vi "Mass Compile - UI - .vi"(7 "Only Check Launcher? (F: Check Entire Product)":bool, 8 "error in (no error)":errorcluster, 10 "Product Folders":path[](array[path]), 11 "Product Name":string) -> (0 "error out":errorcluster, 2 "User Aborted?":bool)   [LabVIEW 2013]
uses:
  <userlib>/_OpenG.lib/appcontrol/appcontrol.llb/Close Generic Object Refnum (Array VI)__ogtk.vi
  <userlib>/_OpenG.lib/array/array.llb/Conditional Auto-Indexing Tunnel (VI-REF)__ogtk.vi
  <userlib>/_OpenG.lib/array/array.llb/Conditional Auto-Indexing Tunnel (Variant)__ogtk.vi
  <userlib>/_OpenG.lib/array/array.llb/Remove Duplicates from 1D Array (String)__ogtk.vi
  <userlib>/_OpenG.lib/array/array.llb/Delete Elements from 1D Array (Variant)__ogtk.vi
  <userlib>/_OpenG.lib/appcontrol/appcontrol.llb/Close Generic Object Refnum (Scalar VI)__ogtk.vi
panel:
  out "Sub-state":string
  out "Slide":u8(slide) scale=0.0..100.0
  out "Elapsed Time":dbl format="%<%H:%M:%S%0u>t"
  in  "abort":bool
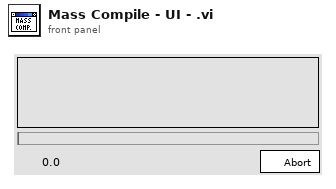
[diagram p1: front panel]
types:
  T1 = cluster{"Current VI's reference":refnum<vi>, "VIs to Recompiled":refnum<vi>[], "Libraries to Recompiled":refnum<vi>[], "Total size":i32, "Current":i32, "Start time":timestamp, "VI Path":path, "Product Folders":path[], "User Aborted":bool}
  T2 = cluster{"Minimum":dbl, "Maximum":dbl, "Increment":dbl, "Minor Incr":dbl, "Start":dbl}
  T3 = enum32{"Invalid", "Standard", "Closed", "Hidden", "Minimized", "Maximized"}
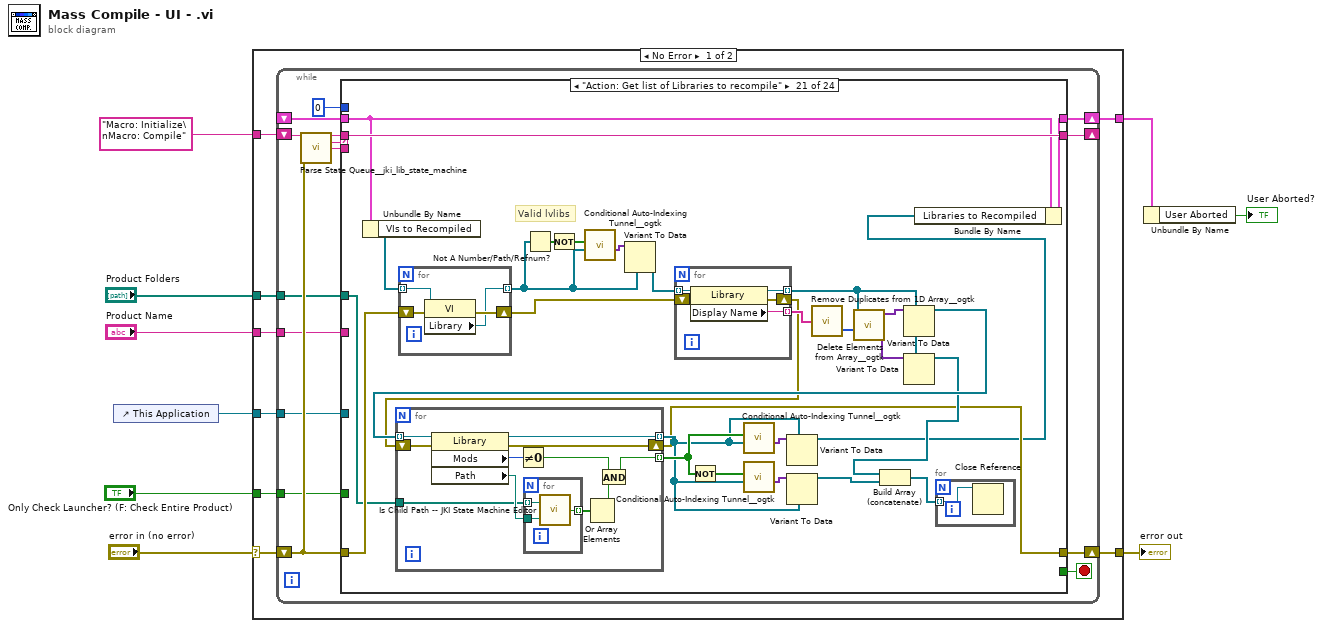
[diagram p0: block diagram]
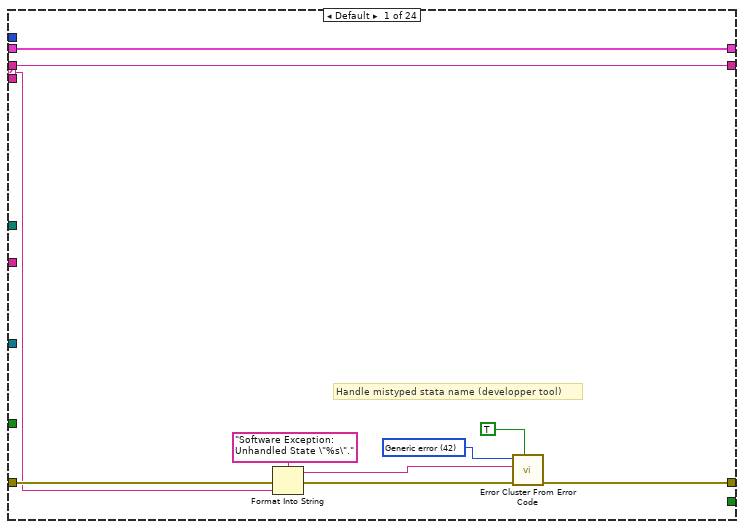
[diagram p2: hidden frame]
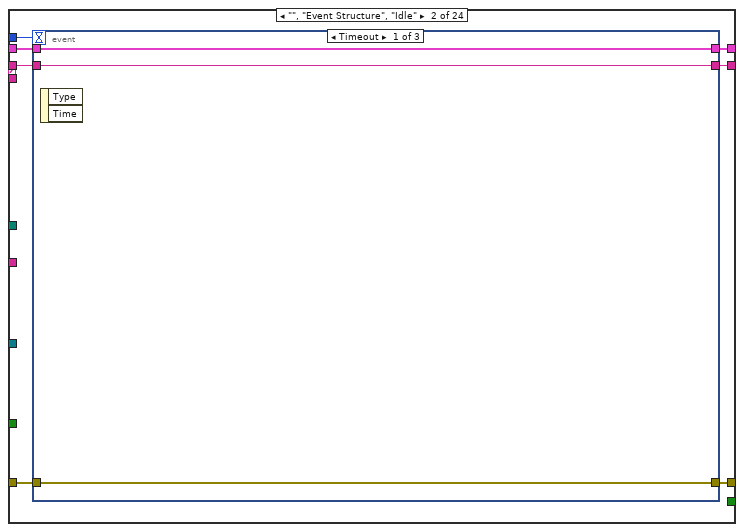
[diagram p3: hidden frame]
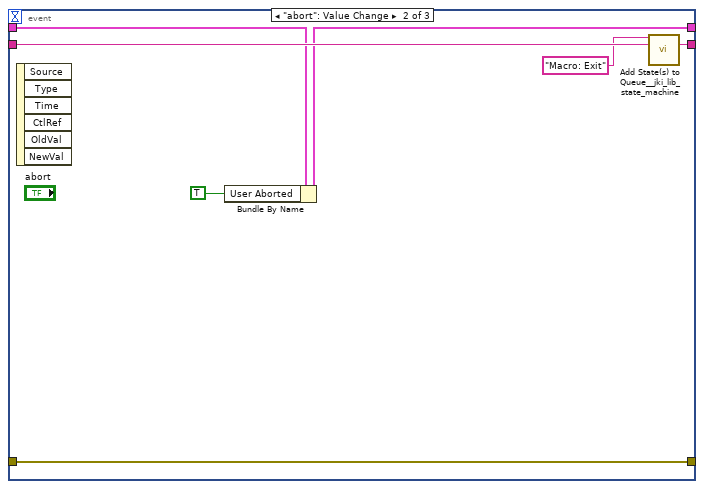
[diagram p4: hidden frame]
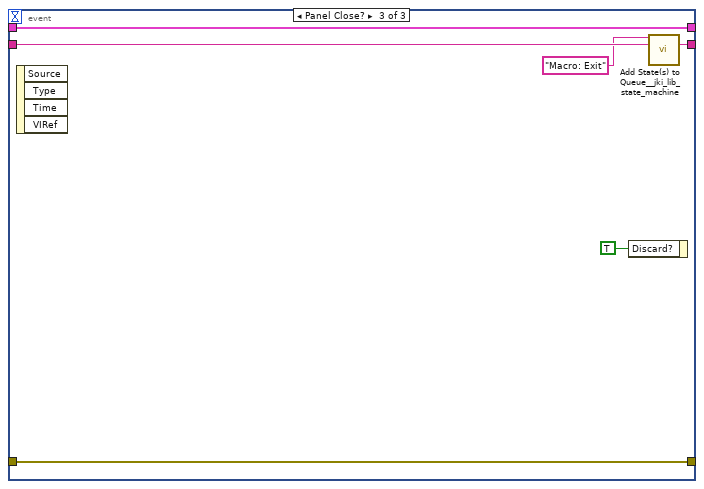
[diagram p5: hidden frame]
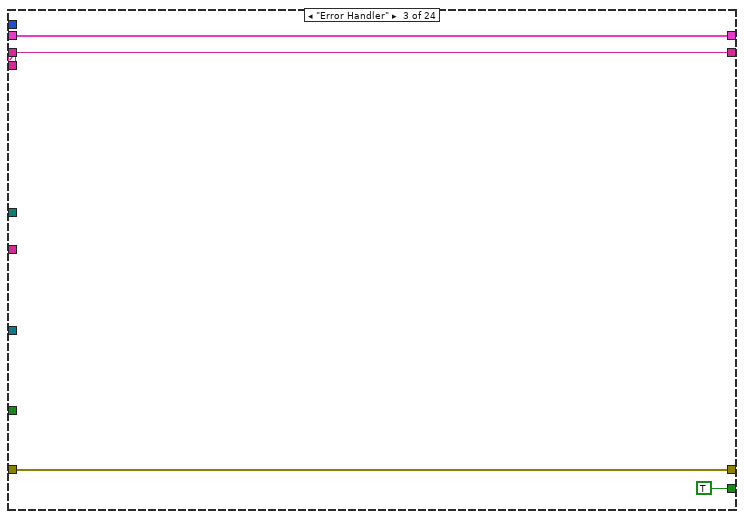
[diagram p6: hidden frame]
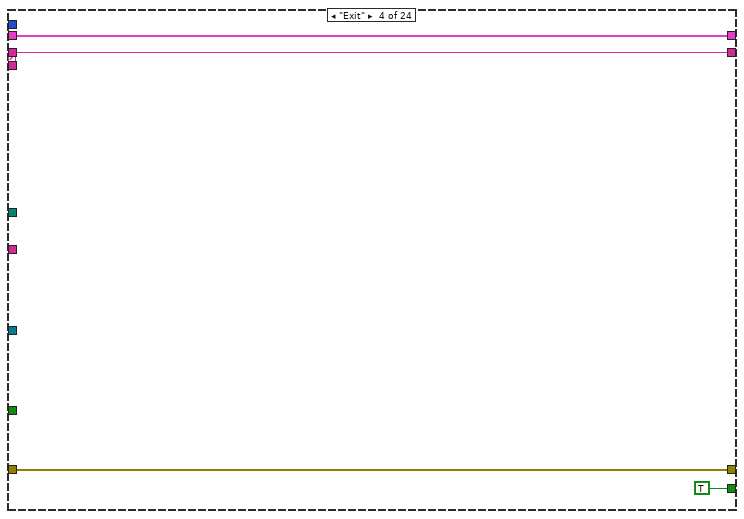
[diagram p7: hidden frame]
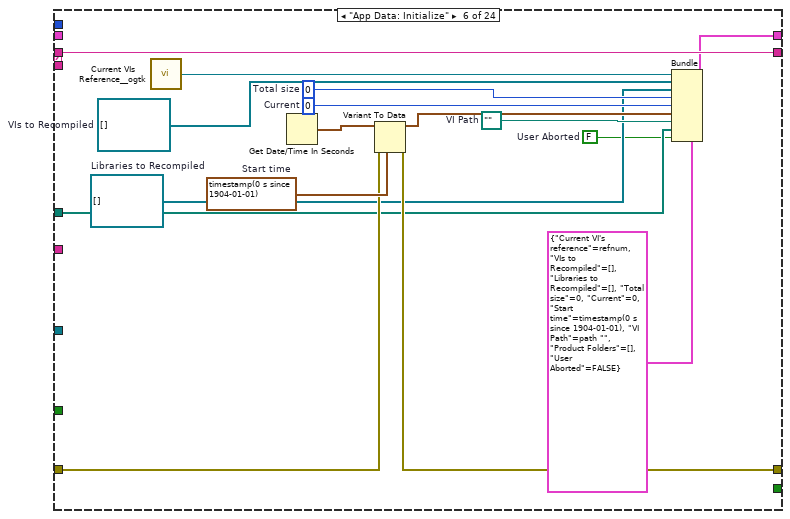
[diagram p9: hidden frame]
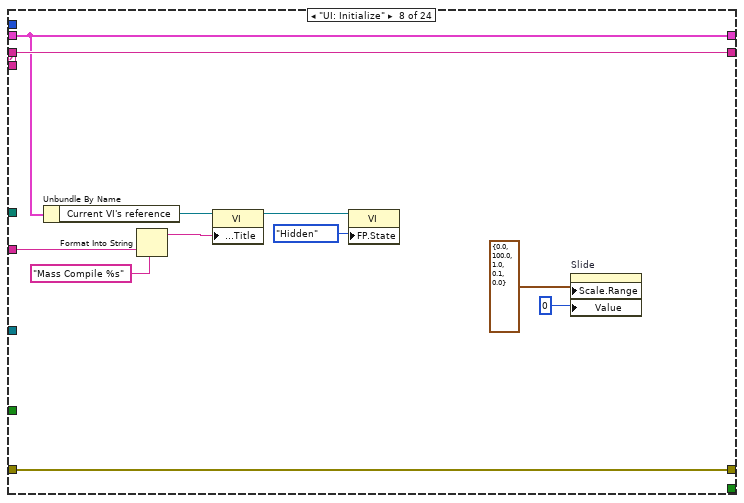
[diagram p11: hidden frame]
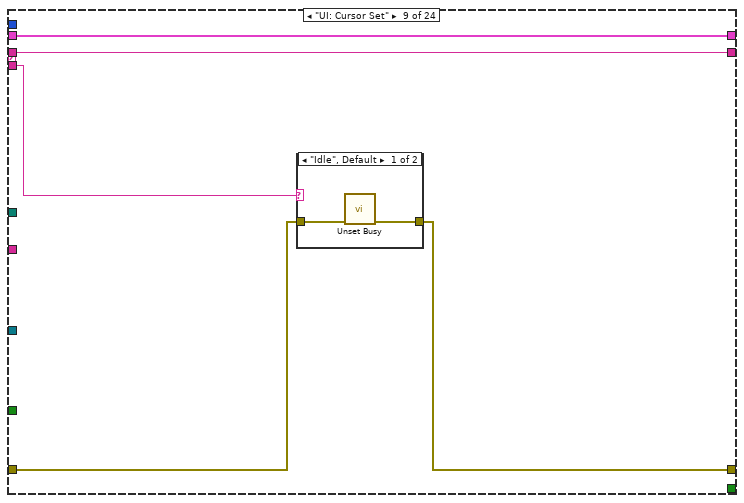
[diagram p12: hidden frame]
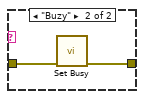
[diagram p13: hidden frame]
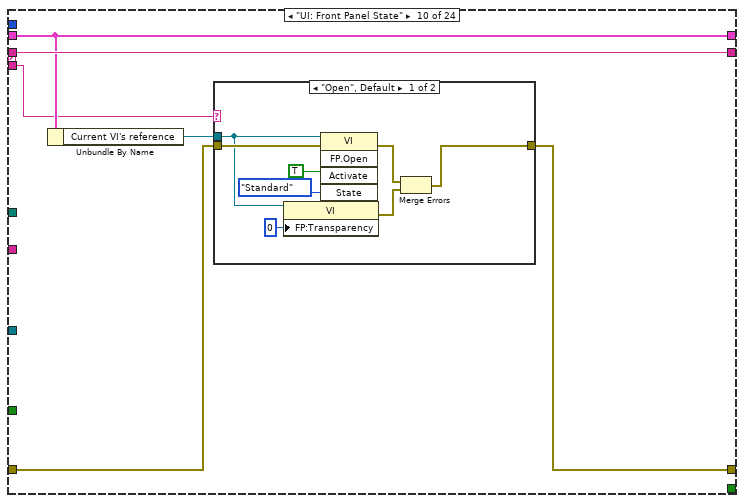
[diagram p14: hidden frame]
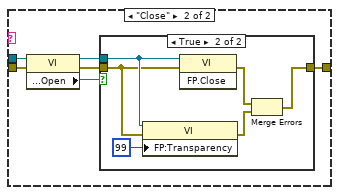
[diagram p15: hidden frame]
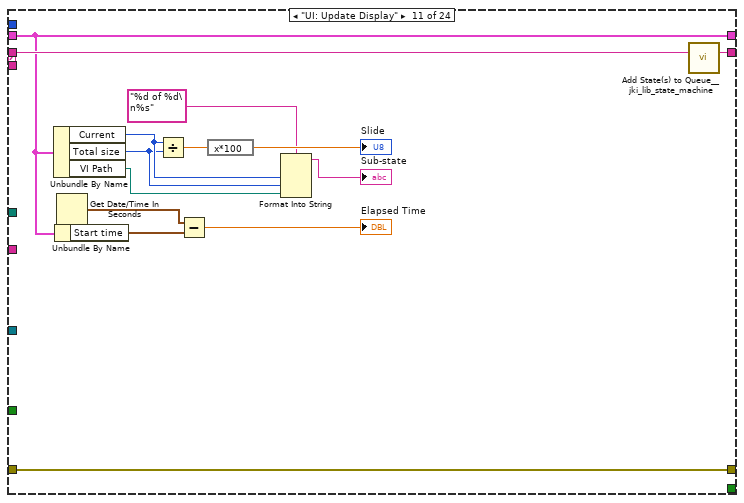
[diagram p17: hidden frame]
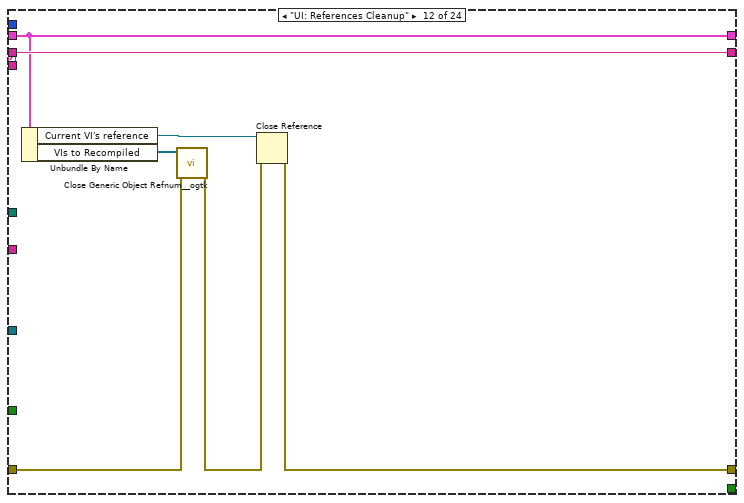
[diagram p18: hidden frame]
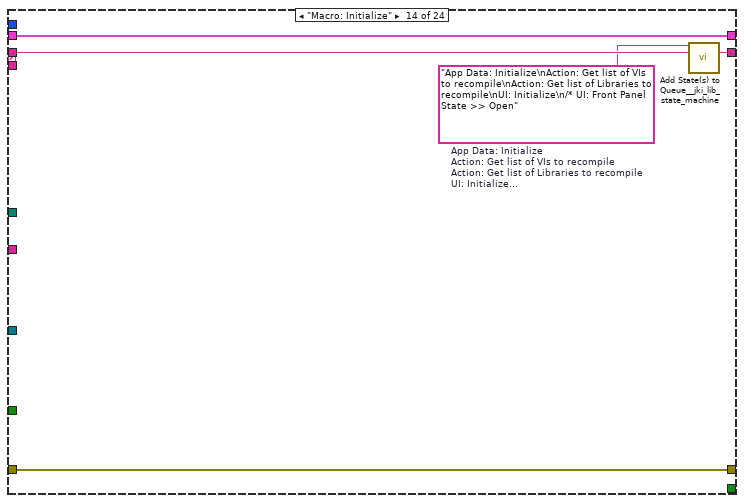
[diagram p20: hidden frame]
diagram:
  n1 = control-ref of="This Application"() -> (w3:refnum<vi>)
  n2 = case shown="No Error" "error in (no error)" {
    selector: "error in (no error)" -> [w14 w365]
    tunnel: "Macro: Initialize\nMacro: Compile" -> [w17 _]
    tunnel: "Product Name" -> [w16 _]
    tunnel: [w15 w365] -> w7
    tunnel: "Product Folders" -> [w13 _]
    tunnel: "Only Check Launcher? (F: Check Entire Product)" -> [w12 _]
    tunnel: w3 -> [w11 _]
    tunnel: [w10 _] -> w2
    frame No Error {
      n3 = while {
        shift-right: [w23] -> w10
        shift-left: _ -> [w28]
        shift-right: [w27] -> w15
        shift-left: w14 -> [w26]
        shift-right: [w25] -> _
        shift-left: w17 -> [w29]
        tunnel: w16 -> [w22]
        tunnel: w13 -> [w20]
        tunnel: w12 -> [w19]
        tunnel: w11 -> [w18]
        stop <- w24 stop-if-true
        n4 = call <vilib>:"Parse State Queue__jki_lib_state_machine.vi"("State Queue"=w29, "Error In (no error)"=w26) -> ("Remaining States"=w31:string, "Current State"=w32:string, "Arguments"=w30:string)  [unwired: 11 in]
        n5 = case shown="\"Action: Get list of Libraries to recompile\"" w32 {
          selector: w32 -> [w36 _ _ _ _ _ _ _ _ _ _ _ _ _ _ _ _ _ _ _ _ _ w332 _]
          tunnel: w31 -> [w35 w49 w69 w73 w76 w92 w95 w106 w111 w121 w156 w163 w166 w171 w190 w201 w204 w209 w219 w239 w299 w329 w354 w359]
          tunnel: w30 -> [_ _ _ _ _ _ _ _ w107 w118 _ _ _ _ _ _ _ _ _ _ _ w327 _ _]
          tunnel: w28 -> [w34 w47 w68 w72 w74 _ w93 w105 w110 w119 w152 w162 w164 w168 w187 w198 w202 w206 w217 w234 w289 w328 w342 w358]
          tunnel: [w38 w46 w67 w71 w75 w82 w94 w96 w108 w116 w148 w160 w165 w169 w188 w199 w203 w207 w218 w231 w272 w325 w351 w356] -> w27
          tunnel: w26 -> [w37 w45 w67 w71 w75 w83 w94 w96 w109 w117 w148 w158 w165 w169 w188 w199 w203 w207 w218 w232 w287 w326 w343 w355]
          tunnel: [w35 w48 w69 w73 w76 w92 w95 w106 w111 w121 w155 w163 w166 w170 w189 w200 w204 w208 w219 w239 w299 w329 w353 w359] -> w25
          tunnel: [_ _ TRUE TRUE _ _ _ _ _ _ _ _ _ _ _ _ _ _ _ _ _ _ _ _] -> w24
          tunnel: [w34 w44 w68 w72 w74 w91 w93 w105 w110 w119 w152 w162 w164 w168 w187 w198 w202 w206 w217 w233 w298 w328 w352 w358] -> w23
          tunnel: w22 -> [_ _ _ _ _ _ _ w98 _ _ _ _ _ _ w182 _ _ _ _ _ _ _ _ _]
          tunnel: 0 -> [_ w43 _ _ _ _ _ _ _ _ _ _ _ _ _ _ _ _ _ _ _ _ _ _]
          tunnel: w20 -> [_ _ _ _ _ w80 _ _ _ _ _ _ _ _ _ _ _ _ _ w229 w277 _ _ _]
          tunnel: w19 -> [_ _ _ _ _ _ _ _ _ _ _ _ _ _ _ _ _ _ _ w220 _ _ _ _]
          tunnel: w18 -> [_ _ _ _ _ _ _ _ _ _ _ _ _ _ _ _ _ _ _ w221 _ _ _ _]
          frame Default {
            w41 = 42 items=["No error", "Argument error", "Memory is full", "Out of zone", "End of file", "File already open", "Generic file I/O error", "File not found", "File permission error", "Disk is full", "Duplicate path", "Too many files open", "System feature not enabled", "Resource file not found", "Cannot add resource", "Resource not found", "Image not found", "Image memory error", "Pen does not exist", "Config type invalid", "Config token not found", "Config parse error", "Config memory error", "Bad external code format", "Bad external code offset", "External code not present", "Null window", "Destroy window error", "Null menu", "Print aborted", "Bad print record", "Print driver error", "Windows error during printing", "Memory error during printing", "Print dialog error", "Generic print error", "Invalid device refnum", "Device not found", "Device parameter error", "Device unit error", "Cannot open device", "Device call aborted", "Generic error", "Cancelled by user", "Object ID too low", "Object ID too high", "Object not in heap", "Unknown heap", "Unknown object (invalid DefProc)", "Unknown object (DefProc not in table)", "Message out of range", "Invalid (null) method", "Unknown message", "Manager call not supported", "Bad address", "Network operation in progress", "Network operation timed out", "Connection is busy", "Network attribute not supported", "Network error", "Address in use", "System out of memory", "Connection aborted", "Connection refused", "Not connected", "Already connected", "Connection closed", "Initialization error (interapplication manager)", "Bad occurrence", "Wait on unbound occurrence handler", "Occurrence queue overflow", "Datalog type conflict", "Unused", "Unrecognized type (interapplication manager)", "Memory corrupt", "Failed to make temporary DLL", "Old CIN version", "Drag socket not found", "Failed to load drop-object", "Failed to register OLE object", "Failed to release OLE object", "Format specifier type mismatch", "Unknown format specifier", "Too few format specifiers", "Too many format specifiers", "Scan failed", "Newer CIN version", "Error converting to variant", "Runtime menu error", "Password tampered", "Variant attribute not found", "Incompatible variant data type", "Event data is not available", "Event Store is not present", "Occurrence is not found", "Event Queue is not created", "Event info is not available", "Refnum passed is NULL", "Error retrieving Class GUID", "Error retrieving CoClass GUID", "Error retrieving TypeLib GUID.", "Bad built application magic bytes.", "Specific driver is different from the specific driver associated with the Logical Name.", "There is no session opened to the class driver.", "Max Error", "MAX - Error with config objects", "MAX - Error loading configuration", "MAX - Group not supported"]
            # "Handle mistyped stata name (developper tool)"
            n6 = Format Into String(format string="Software Exception: Unhandled State \"%s\"." ("message"), error in=w37, w36) -> (resulting string=w40:string, error out=w39:errorcluster)  [unwired: 1 in]
            n7 = call <vilib>:"Error Cluster From Error Code.vi"("show call chain? (False)"=TRUE, "error in (no error)"=w39, "error message (\"\")"=w40, "error code (0)"=w41) -> ("error out"=w38:errorcluster)  [unwired: 5 in]
          }
          frame "", "Event Structure", "Idle" {
            n8 = event shown="[0] Timeout" {
              selector: _ -> [_ _ _]
              dyn-events: _ -> [_ _ _]
              timeout: w43 -> [_ _ _]
              tunnel: w49 -> [w52 w59 w65]
              tunnel: [w52 w58 w64] -> w48
              tunnel: w47 -> [w50 w56 w62]
              tunnel: [w51 w57 w63] -> w46
              tunnel: w45 -> [w51 w57 w63]
              tunnel: [w50 w54 w62] -> w44
              event Timeout {
                n9 = event-data() -> ()  [unwired: 1 in, 2 out]
              }
              event "abort": Value Change {
                n10 = event-data() -> ()  [unwired: 1 in, 6 out]
                n11 = Bundle By Name(cluster=w56, "User Aborted"=TRUE) -> (w54:T1)
                n12 = call <vilib>:"Add State(s) to Queue__jki_lib_state_machine.vi"("State(s) in Front (\"\")"="Macro: Exit", "State(s) in (\"\")"=w59) -> ("States Out"=w58:string)  [unwired: 13 in]
              }
              event Panel Close? {
                n13 = event-data() -> ()  [unwired: 1 in, 4 out]
                n14 = event-data("Discard?"=TRUE) -> ()  [unwired: 1 in, 1 out]
                n15 = call <vilib>:"Add State(s) to Queue__jki_lib_state_machine.vi"("State(s) in Front (\"\")"="Macro: Exit", "State(s) in (\"\")"=w65) -> ("States Out"=w64:string)  [unwired: 13 in]
              }
            }
          }
          frame "Error Handler" {
          }
          frame "Exit" {
          }
          frame "---------- App Data ----------" {
          }
          frame "App Data: Initialize" {
            w77 = FALSE  # User Aborted
            w79 = refnum<vi>[] []  # Libraries to Recompiled
            w81 = path ""  # VI Path
            w86 = timestamp(0 s since 1904-01-01)  # Start time
            w87 = 0  # Current
            w88 = 0  # Total size
            w89 = refnum<vi>[] []  # VIs to Recompiled
            n16 = call <userlib>:"Current VIs Reference__ogtk.vi"() -> ("Current VI's reference"=w90:refnum<vi>)  [unwired: 5 in]
            n17 = Get Date/Time In Seconds() -> (seconds since 1Jan1904=w85:timestamp)
            n18 = Variant To Data(error in=w83, type=w86, Variant=w85) -> (data=w84:timestamp, error out=w82:errorcluster)
            n19 = Bundle(cluster=T1 {"Current VI's reference"=refnum, "VIs to Recompiled"=[], "Libraries to Recompiled"=[], "Total size"=0, "Current"=0, "Start time"=timestamp(0 s since 1904-01-01), "VI Path"=path "", "Product Folders"=[], "User Aborted"=FALSE}, "Current VI's reference"=w90, "VIs to Recompiled"=w89, "Libraries to Recompiled"=w79, "Total size"=w88, "Current"=w87, "Start time"=w84, "VI Path"=w81, "Product Folders"=w80, "User Aborted"=w77) -> (w91:T1)
          }
          frame "---------- UI ----------" {
          }
          frame "UI: Initialize" {
            n20 = Unbundle By Name(w105) -> ("Current VI's reference"=w101:refnum<vi>)
            n21 = Format Into String(format string="Mass Compile %s", w98) -> (resulting string=w97:string)  [unwired: 2 in, 1 out]
            n22 = property class="VI"(reference=w101, "Front Panel.Title"=w97) -> (reference out=w100:refnum<vi>)  [unwired: 1 in, 1 out]
            n23 = property class="VI"(reference=w100, "FP.State"=T3."Hidden" ("Front Panel Window:State")) -> ()  [unwired: 1 in, 2 out]
            n24 = property on="Slide" class="Slide (strict)"("Scale.Range"=T2 {"Minimum"=0.0, "Maximum"=100.0, "Increment"=1.0, "Minor Incr"=0.1, "Start"=0.0}, "Value"=0) -> ()  [unwired: 2 in, 2 out]
          }
          frame "UI: Cursor Set" {
            n25 = case shown="\"Idle\", Default" w107 {
              tunnel: w109 -> [w113 w115]
              tunnel: [w112 w114] -> w108
              frame "Idle", Default {
                n26 = call <vilib>:"Unset Busy.vi"("error in (no error)"=w113) -> ("error out"=w112:errorcluster)  [unwired: 10 in]
              }
              frame "Buzy" {
                n27 = call <vilib>:"Set Busy.vi"("error in (no error)"=w115) -> ("error out"=w114:errorcluster)  [unwired: 9 in, 1 out]
              }
            }
          }
          frame "UI: Front Panel State" {
            n28 = Unbundle By Name(w119) -> ("Current VI's reference"=w120:refnum<vi>)
            n29 = case shown="\"Open\", Default" w118 {
              tunnel: w120 -> [w125 w134]
              tunnel: w117 -> [w127 w133]
              tunnel: [w122 w135] -> w116
              frame "Open", Default {
                n30 = property class="VI"(reference=w125, "FP:Transparency"=u8 0 ("Front Panel Window:Transparency")) -> (error out=w124:errorcluster)  [unwired: 1 in, 1 out]
                n31 = invoke class="VI" method="FP.Open"(reference=w125, error in=w127, "Activate"=TRUE, "State"=T3."Standard") -> (error out=w123:errorcluster)  [unwired: 1 in, 4 out]
                n32 = Merge Errors(w123, w124) -> (w122:errorcluster)
              }
              frame "Close" {
                n33 = property class="VI"(reference=w134, error in=w133) -> (reference out=w132:refnum<vi>, error out=w131:errorcluster, "Front Panel.Open"=w130:bool)
                n34 = case shown="True" w130 {
                  tunnel: w132 -> [_ w142]
                  tunnel: w131 -> [w136 w140]
                  tunnel: [w136 w137] -> w135
                  frame False {
                  }
                  frame True {
                    n35 = property class="VI"(reference=w142, error in=w140, "FP:Transparency"=u8 99 ("Front Panel Window:Transparency")) -> (error out=w138:errorcluster)  [unwired: 1 out]
                    n36 = invoke class="VI" method="FP.Close"(reference=w142, error in=w140) -> (error out=w139:errorcluster)  [unwired: 1 in, 2 out]
                    n37 = Merge Errors(w139, w138) -> (w137:errorcluster)
                  }
                }
              }
            }
          }
          frame "UI: Update Display" {
            n38 = Unbundle By Name(w152) -> ("Current"=w146:i32, "Total size"=w145:i32, "VI Path"=w144:path)
            n39 = Unbundle By Name(w152) -> ("Start time"=w151:timestamp)
            n40 = Get Date/Time In Seconds() -> (seconds since 1Jan1904=w150:timestamp)
            n41 = Divide(x=w146, y=w145) -> (x/y=w154:dbl)
            n42 = Subtract(x=w150, y=w151) -> (x-y=→"Elapsed Time":dbl)
            n43 = expression code="x*100"(w154) -> (→"Slide":dbl)
            n44 = Format Into String(format string="%d of %d\n%s", w146, w145, w144) -> (resulting string=→"Sub-state":string)  [unwired: 2 in, 1 out]
            n45 = call <vilib>:"Add State(s) to Queue__jki_lib_state_machine.vi"("State(s) in (\"\")"=w156) -> ("States Out"=w155:string)  [unwired: 14 in]
          }
          frame "UI: References Cleanup" {
            n46 = Unbundle By Name(w162) -> ("Current VI's reference"=w161:refnum<vi>, "VIs to Recompiled"=w159:refnum<vi>[])
            n47 = call-poly <userlib>:"Close Generic Object Refnum__ogtk.vi"("error in (no error)"=w158, "Gen Refnum Array"=w159) -> ("error out"=w157:errorcluster)  [unwired: 8 in, 1 out]
            n48 = Close Reference(reference=w161, error in (no error)=w157) -> (error out=w160:errorcluster)
          }
          frame "---------- Macro ----------" {
          }
          frame "Macro: Initialize" {
            w167 = "App Data: Initialize\nAction: Get list of VIs to recompile\nAction: Get list of Libraries to recompile\nUI: Initialize\n/* UI: Front Panel State >> Open"  # App Data: Initialize Action: Get list of VIs to recompile Action: Get list of Libraries to recompile UI: Initialize /* UI: Front Panel State >> Open
            n49 = call <vilib>:"Add State(s) to Queue__jki_lib_state_machine.vi"("State(s) in Front (\"\")"=w167, "State(s) in (\"\")"=w171) -> ("States Out"=w170:string)  [unwired: 13 in]
          }
          frame "Macro: Compile" {
            (unwired) "<color=red>You appears to be running the %s for the first time after installation. \nYou should mass compile the %s before you can use it effectively.</color>"
            w184 = "UI: Front Panel State >> Open\nAction: Set LLB Caching >> On\nAction: Mass Compile\nAction: Mass Compile Libraries\nAction: Set LLB Caching >> Off\nMacro: Exit"  # UI: Front Panel State >> Open Action: Set LLB Caching >> On Action: Mass Compile Action: Mass Compile Libraries Action: Set LLB Caching >> Off Macro: Exit
            n50 = Unbundle By Name(w187) -> ("Libraries to Recompiled"=w174:refnum<vi>[], "VIs to Recompiled"=w176:refnum<vi>[])
            n51 = property class="App"() -> ("App.Version"=w177:string)  [unwired: 2 in, 2 out]
            n52 = Empty Array?(array=w174) -> (empty?=w175:bool)
            n53 = Empty Array?(array=w176) -> (empty?=w173:bool)
            n54 = And(x=w175, y=w173) -> (x .and. y?=w172:bool)
            n55 = Format Into String(format string="This appears to be the first time you have run %s since it was installed.  %s will now resave itself in LabVIEW %s for maximum performance.", w182, w182, w177) -> (resulting string=w181:string)  [unwired: 2 in, 1 out]
            n56 = Not(x=w172) -> (.not. x?=w178:bool)
            n57 = case "Need to recompile?" shown="True" w178 {
              selector: w178 -> [w191 _]
              tunnel: w182 -> [_ _]
              tunnel: w181 -> [_ w196]
              tunnel: [w191 w192] -> w180
              frame False {
              }
              frame True {
                n58 = Two Button Dialog(message=w196, 1:"Cancel" ("F button name (\"Cancel\")"), 2:"OK" ("T button name (\"OK\")")) -> (T button?=w193:bool)
                n59 = Not(x=w193) -> (.not. x?=w192:bool)
              }
            }
            n60 = Compound Arithmetic op=OR(w172, w180) -> (w179:bool)
            n61 = Select(t="Macro: Exit", s=w179, f=w184) -> (s? t:f=w185:string)
            n62 = call <vilib>:"Add State(s) to Queue__jki_lib_state_machine.vi"("State(s) in Front (\"\")"=w185, "State(s) in (\"\")"=w190) -> ("States Out"=w189:string)  [unwired: 13 in]
          }
          frame "Macro: Exit" {
            n63 = call <vilib>:"Add State(s) to Queue__jki_lib_state_machine.vi"("State(s) in Front (\"\")"="Condition: Check for Panel Close at Exit\nUI: References Cleanup\nExit", "State(s) in (\"\")"=w201) -> ("States Out"=w200:string)  [unwired: 13 in]
          }
          frame "---------- Condition ----------" {
          }
          frame "Condition: Check for Panel Close at Exit" {
            n64 = stacked-sequence {
              tunnel: [w216] -> w205
              frame #0 {
                n65 = Call Chain() -> (call chain=w212:string[])
                n66 = Index Array(array=w212, index=1 ("Index")) -> (element=w211:string)
                n67 = Empty String/Path?(string/path=w211) -> (empty?=w210:bool)
                n68 = Select(t="", s=w210, f="UI: Front Panel State >> Close") -> (s? t:f=w216:string)
              }
            }
            n69 = call <vilib>:"Add State(s) to Queue__jki_lib_state_machine.vi"("State(s) in Front (\"\")"=w205, "State(s) in (\"\")"=w209) -> ("States Out"=w208:string)  [unwired: 13 in]
          }
          frame "---------- Action ----------" {
          }
          frame "Action: Get list of VIs to recompile" {
            n70 = case shown="False" w220 {
              tunnel: w232 -> [w244 w250]
              tunnel: [w243 w247] -> w226
              tunnel: [w242 w251] -> w225
              tunnel: [w241 w249] -> w223
              tunnel: w221 -> [w240 w251]
              frame False {
                n71 = property class="App"(reference=w240, error in=w244) -> (reference out=w242:refnum<vi>, error out=w241:errorcluster, "App.AllSysVIs"=w246:string[], "App.AllVIs"=w245:string[])
                n72 = Build Array (concatenate)(w246, w245) -> (w243:string[])
              }
              frame True {
                n73 = property class="VI"(error in=w250) -> (error out=w249:errorcluster, "Name"=w248:string)  [unwired: 1 in, 1 out]
                n74 = Build Array(w248) -> (w247:string[])
              }
            }
            n75 = for {
              tunnel: w226 -> [w256] mode=indexing
              tunnel: w225 -> [w255]
              tunnel: [w254] -> w224 mode=indexing
              shift-right: [w252] -> w222
              shift-left: w223 -> [w253]
              n76 = Open VI Reference(application reference (local)=w255, vi path=w256, error in (no error)=w253) -> (vi reference=w254:refnum<vi>, error out=w252:errorcluster)  [unwired: 3 in]
            }
            n77 = for {
              shift-right: [w266] -> w235
              shift-left: w222 -> [w257]
              tunnel: [w259] -> w228 mode=indexing
              tunnel: [w265] -> w237 mode=indexing
              tunnel: w229 -> [w263]
              tunnel: w224 -> [w258] mode=indexing
              n78 = property class="VI"(reference=w258, error in=w257) -> (reference out=w265:refnum<vi>, error out=w266:errorcluster, "Mods.VI"=w267:u32, "Path"=w264:path)
              n79 = for {
                tunnel: w264 -> [w270]
                tunnel: w263 -> [w269] mode=indexing
                tunnel: [w268] -> w262 mode=indexing
                n80 = call "Is Child Path -- JKI State Machine Editor.vi"("Path"=w270, "Parent Directory"=w269) -> ("is Child Path?"=w268:bool)
              }
              n81 = Not Equal To 0?(x=w267) -> (x != 0?=w260:bool)
              n82 = Or Array Elements(Boolean array=w262) -> (logical OR=w261:bool)
              n83 = And(x=w260, y=w261) -> (x .and. y?=w259:bool)
            }
            n84 = Not(x=w228) -> (.not. x?=w238:bool[])
            n85 = call-poly <userlib>:"Conditional Auto-Indexing Tunnel__ogtk.vi"("Array in"=w237, "Elements to keep"=w228) -> ("Filtered Array out"=w230:refnum<vi>[])  [unwired: 5 in]
            n86 = call-poly <userlib>:"Conditional Auto-Indexing Tunnel__ogtk.vi"("Array in"=w237, "Elements to keep"=w238) -> ("Filtered Array out"=w236:refnum<vi>[])  [unwired: 5 in]
            n87 = call-poly <userlib>:"Close Generic Object Refnum__ogtk.vi"("error in (no error)"=w235, "Gen Refnum Array"=w236) -> ("error out"=w231:errorcluster)  [unwired: 8 in, 1 out]
            n88 = Array Size(array=w230) -> (size(s)=w227:i32)
            n89 = Bundle By Name(cluster=w234, "VIs to Recompiled"=w230, "Total size"=w227) -> (w233:T1)
          }
          frame "Action: Get list of Libraries to recompile" {
            # "Valid lvlibs"
            n90 = Unbundle By Name(w289) -> ("VIs to Recompiled"=w288:refnum<vi>[])
            n91 = for {
              shift-right: [w323] -> w284
              shift-left: w287 -> [w321]
              tunnel: [w320] -> w286 mode=indexing
              tunnel: w288 -> [w322] mode=indexing
              n92 = property class="VI"(reference=w322, error in=w321) -> (error out=w323:errorcluster, "Library"=w320:refnum<vi>)  [unwired: 1 out]
            }
            n93 = Not A Number/Path/Refnum?(number/path/refnum=w286) -> (NaN/Path/Refnum?=w297:bool[])
            n94 = Not(x=w297) -> (.not. x?=w296:bool[])
            n95 = call-poly <userlib>:"Conditional Auto-Indexing Tunnel__ogtk.vi"("Array in"=w286, "Elements to keep"=w296) -> ("Filtered Array out"=w295:variant[])  [unwired: 5 in]
            n96 = Variant To Data(type=w286, Variant=w295) -> (data=w285:refnum<vi>[])  [unwired: 1 in, 1 out]
            n97 = for {
              tunnel: w285 -> [w304] mode=indexing
              tunnel: [w303] -> w278 mode=indexing
              tunnel: [w301] -> w283 mode=indexing
              shift-right: [w300] -> w273
              shift-left: w284 -> [w302]
              n98 = property class="Library"(reference=w304, error in=w302) -> (reference out=w303:refnum<vi>, error out=w300:errorcluster, "Display Name"=w301:string)
            }
            n99 = call-poly <userlib>:"Remove Duplicates from 1D Array__ogtk.vi"("Input Array"=w283) -> ("indices of removed elements"=w282:i32[])  [unwired: 1 out]
            n100 = call-poly <userlib>:"Delete Elements from Array__ogtk.vi"("indices"=w282, "array"=w278) -> ("deleted elements"=w279:variant[], "array w/ subset deleted"=w281:variant[])  [unwired: 8 in]
            n101 = Variant To Data(type=w278, Variant=w281) -> (data=w280:refnum<vi>[])  [unwired: 1 in, 1 out]
            n102 = for {
              tunnel: w280 -> [w316] mode=indexing
              tunnel: [w308] -> w293 mode=indexing
              tunnel: [w314] -> w290 mode=indexing
              tunnel: w277 -> [w310]
              shift-right: [w307] -> w272
              shift-left: w273 -> [w306]
              n103 = property class="Library"(reference=w316, error in=w306) -> (reference out=w314:refnum<vi>, error out=w307:errorcluster, "Mods"=w315:i32, "Path"=w311:path)
              n104 = Not Equal To 0?(x=w315) -> (x != 0?=w309:bool)
              n105 = for {
                tunnel: w311 -> [w319]
                tunnel: w310 -> [w318] mode=indexing
                tunnel: [w317] -> w313 mode=indexing
                n106 = call "Is Child Path -- JKI State Machine Editor.vi"("Path"=w319, "Parent Directory"=w318) -> ("is Child Path?"=w317:bool)
              }
              n107 = Or Array Elements(Boolean array=w313) -> (logical OR=w312:bool)
              n108 = And(x=w309, y=w312) -> (x .and. y?=w308:bool)
            }
            n109 = Not(x=w293) -> (.not. x?=w294:bool[])
            n110 = call-poly <userlib>:"Conditional Auto-Indexing Tunnel__ogtk.vi"("Array in"=w290, "Elements to keep"=w293) -> ("Filtered Array out"=w292:variant[])  [unwired: 5 in]
            n111 = call-poly <userlib>:"Conditional Auto-Indexing Tunnel__ogtk.vi"("Array in"=w290, "Elements to keep"=w294) -> ("Filtered Array out"=w291:variant[])  [unwired: 5 in]
            n112 = Variant To Data(type=w290, Variant=w292) -> (data=w271:refnum<vi>[])  [unwired: 1 in, 1 out]
            n113 = Variant To Data(type=w290, Variant=w291) -> (data=w276:refnum<vi>[])  [unwired: 1 in, 1 out]
            n114 = Variant To Data(type=w278, Variant=w279) -> (data=w274:refnum<vi>[])  [unwired: 1 in, 1 out]
            n115 = Build Array (concatenate)(w274, w276) -> (w275:refnum<vi>[])
            n116 = Bundle By Name(cluster=w289, "Libraries to Recompiled"=w271) -> (w298:T1)
            n117 = for {
              tunnel: w275 -> [w305] mode=indexing
              n118 = Close Reference(reference=w305) -> ()  [unwired: 1 in, 1 out]
            }
          }
          frame "Action: Set LLB Caching" {
            n119 = case shown="\"On\", \"True\"" w327 {
              tunnel: [FALSE TRUE] -> w324
              frame "False", "Off", Default {
              }
              frame "On", "True" {
              }
            }
            n120 = call "Proxy - Dist Set LLB Caching.vi"("error in (no error)"=w326, "enable?"=w324) -> ("error out"=w325:errorcluster)  [unwired: 9 in]
          }
          frame "Action: Mass Compile" {
            w334 = "UI: Update Display\nIdle"
            n121 = Unbundle By Name(w342) -> ("VIs to Recompiled"=w350:refnum<vi>[])
            n122 = Unbundle By Name(w342) -> ("Total size"=w340:i32)
            n123 = Delete From Array(array=w350, index=0) -> (deleted portion=w344:refnum<vi>, array with subset deleted=w341:refnum<vi>[])  [unwired: 1 in]
            n124 = Empty Array?(array=w341) -> (empty?=w348:bool)
            n125 = property class="VI"(reference=w344, error in=w343) -> (reference out=w338:refnum<vi>, error out=w335:errorcluster, "Path"=w336:path)
            n126 = Array Size(array=w341) -> (size(s)=w339:i32)
            n127 = Subtract(x=w340, y=w339) -> (x-y=w337:i32)
            n128 = invoke class="VI" method="Save.Instrument"(reference=w338, error in=w335) -> (reference out=w345:refnum<vi>, error out=w346:errorcluster)  [unwired: 4 in, 4 out]
            n129 = call <vilib>:"Add State(s) to Queue__jki_lib_state_machine.vi"("State(s) in Front (\"\")"=w334, "State(s) in (\"\")"=w332) -> ("States Out"=w333:string)  [unwired: 13 in]
            n130 = Select(t=w334, s=w348, f=w333) -> (s? t:f=w347:string)
            n131 = call-poly <userlib>:"Close Generic Object Refnum__ogtk.vi"("error in (no error)"=w346, "VI Refnum"=w345) -> ("error out"=w351:errorcluster)  [unwired: 8 in, 1 out]
            n132 = Bundle By Name(cluster=w342, "VIs to Recompiled"=w341, "Current"=w337, "VI Path"=w336) -> (w352:T1)
            n133 = call <vilib>:"Add State(s) to Queue__jki_lib_state_machine.vi"("State(s) in Front (\"\")"=w347, "State(s) in (\"\")"=w354) -> ("States Out"=w353:string)  [unwired: 13 in]
          }
          frame "Action: Mass Compile Libraries" {
            n134 = Unbundle By Name(w358) -> ("Libraries to Recompiled"=w357:refnum<vi>[])
            n135 = for {
              tunnel: w357 -> [w364] mode=indexing
              shift-right: [w361] -> w356
              shift-left: w355 -> [w360]
              n136 = invoke class="Library" method="Save"(reference=w364, error in=w360) -> (reference out=w363:refnum<vi>, error out=w362:errorcluster)  [unwired: 2 in, 2 out]
              n137 = Close Reference(reference=w363, error in (no error)=w362) -> (error out=w361:errorcluster)
            }
          }
        }
      }
    }
    frame Error {
    }
  }
  "error out" <- w7
  n138 = Unbundle By Name(w2) -> ("User Aborted"=→"User Aborted?":bool)
